vi "FTP_STOR2.vi"(0 "error in":errorcluster, 1 "File to send":string, 2 "Remote Path":string, 3 "connection ID":refnum<k5>) -> (4 "Good Reply?":bool, 5 "error out":errorcluster, 7 "reply string":string, 8 "connection ID out":refnum<k5>)   [LabVIEW 2012]
panel:
  in  "chunk size (4096)":i32=4096
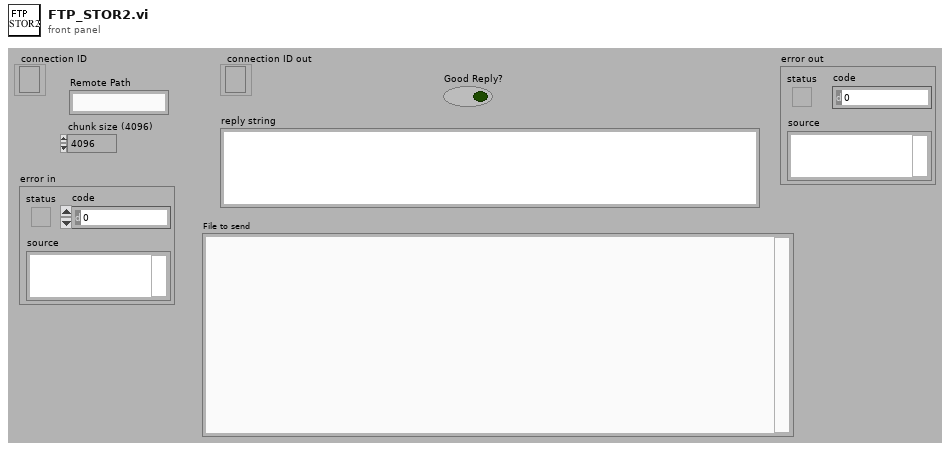
[diagram p1: front panel]
types:
  T1 = enum16{"unknown", "100 + Prelim", "200 + ", "300 + Intermed", "400 - Transient", "500 - Permanent"}
  T2 = cluster{"passive address":string, "passive port":u16}
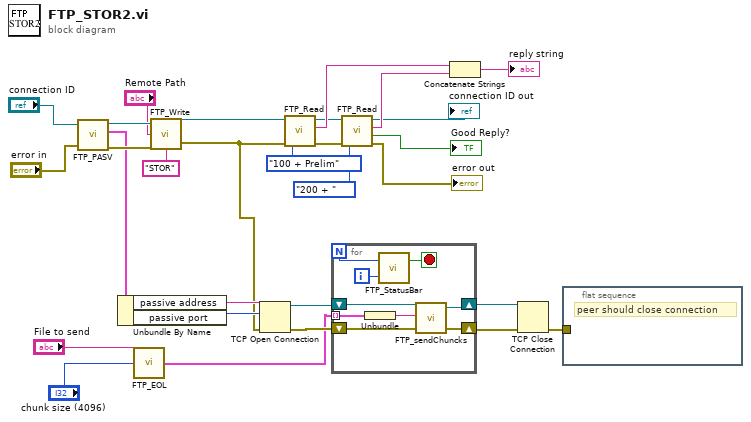
[diagram p0: block diagram]
diagram:
  n1 = call <userlib>:"FTP_PASV.vi"("connection ID"="connection ID", "error in"="error in") -> ("connection ID out"=w26:refnum<k5>, "Passive Port"=w22:T2, "error out"=w25:errorcluster)  [unwired: 2 out]
  n2 = Unbundle By Name(w22) -> ("passive address"=w23:string, "passive port"=w24:u16)
  n3 = call <userlib>:"FTP_EOL.vi"("chunk size (4096)"="chunk size (4096)", "String"="File to send") -> ("chuncks"=w1:cluster{"result string":string}[])  [unwired: 1 out]
  n4 = call <userlib>:"FTP_Write.vi"("Cmd"="STOR", "error in"=w25, "data"="Remote Path", "connection ID in"=w26) -> ("error out"=w12:errorcluster, "connection ID out"=w13:refnum<k5>)
  n5 = TCP Open Connection(address=w23, remote port or service name=w24, error in (no error)=w12) -> (connection ID=w7:refnum<k5>, error out=w6:errorcluster)  [unwired: 2 out]
  n6 = call <userlib>:"FTP_Read.vi"("error In"=w12, "expected class"=T1."100 + Prelim", "connection ID"=w13) -> ("error out"=w19:errorcluster, "reply string"=w18:string, "connection ID out"=w15:refnum<k5>)  [unwired: 2 out]
  n7 = for {
    N -> [w31]
    tunnel: w1 -> [w34] mode=indexing
    shift-right: [w35] -> w5
    shift-left: w7 -> [w38]
    shift-right: [w36] -> w4
    shift-left: w6 -> [w37]
    i -> [w32]
    stop <- w30 stop-if-true
    n8 = Unbundle(w34) -> ("result string"=w33:string)
    n9 = call <userlib>:"FTP_StatusBar.vi"("i"=w32, "N"=w31) -> ("Stop out"=w30:bool)  [unwired: 1 in]
    n10 = call <userlib>:"FTP_sendChuncks.vi"("error in (no error)"=w37, "data in"=w33, "connection ID"=w38) -> ("error out"=w36:errorcluster, "connection ID out"=w35:refnum<k5>)  [unwired: 1 out]
  }
  n11 = call <userlib>:"FTP_Read.vi"("error In"=w19, "expected class"=T1."200 + ", "connection ID"=w15) -> ("error out"=→"error out":errorcluster, "Good Reply?"=→"Good Reply?":bool, "reply string"=w17:string, "connection ID out"=→"connection ID out":refnum<k5>)  [unwired: 1 out]
  n12 = Concatenate Strings(w18, w17) -> (→"reply string":string)
  n13 = TCP Close Connection(connection ID=w5, error in (no error)=w4) -> (error out=w21:errorcluster)  [unwired: 2 out]
  n14 = flat-sequence {
    tunnel: w21 -> [_]
    frame #0 {
      # "peer should close connection"
    }
  }
